vi "BM0211 Image property read write.vi"(9 "Read write":enum16{"write", "Read"}(ring)=enum."Read", 11 "IN":T1(array[cluster])) -> (0 "error out":errorcluster, 3 "Out":T1(array[cluster]))   [LabVIEW 2015]
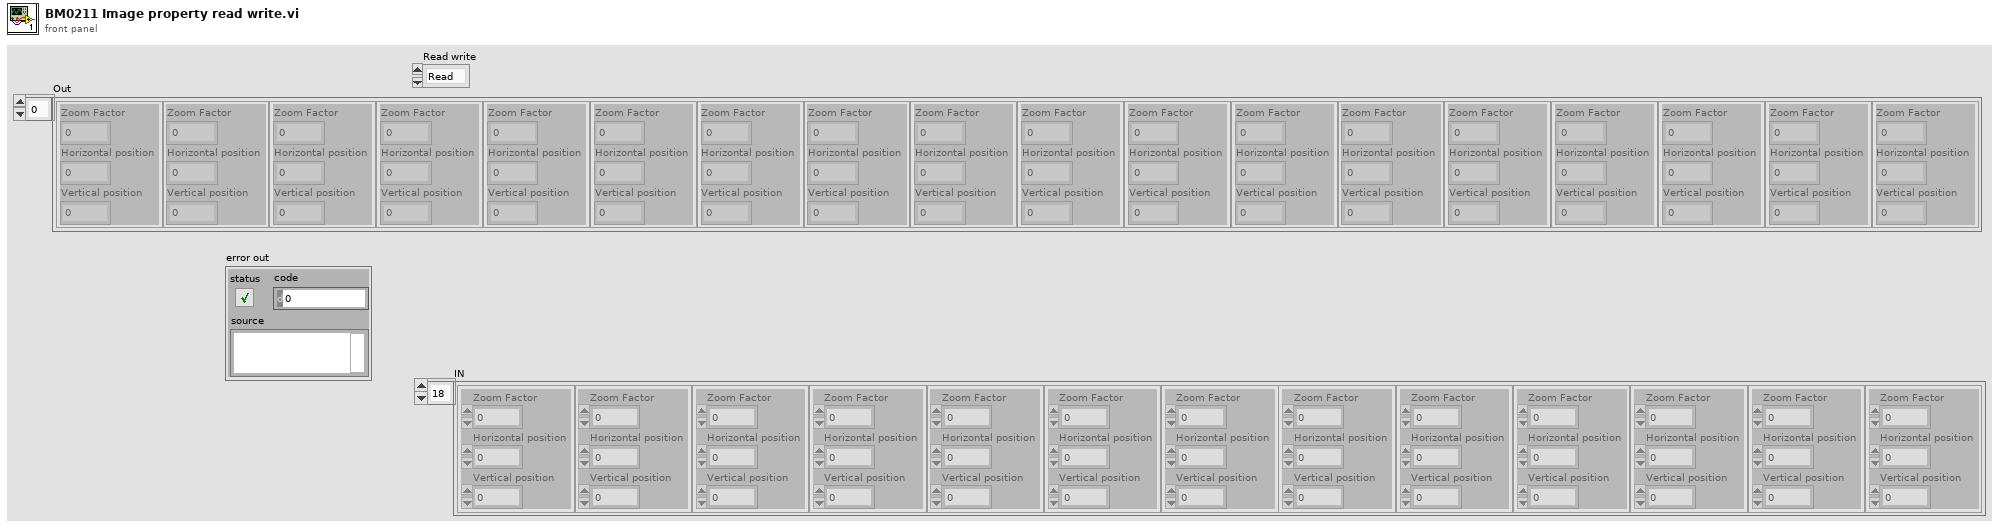
[diagram p1: front panel]
types:
  T1 = cluster{"Zoom Factor":sgl, "Horizontal position":sgl, "Vertical position":sgl}[]
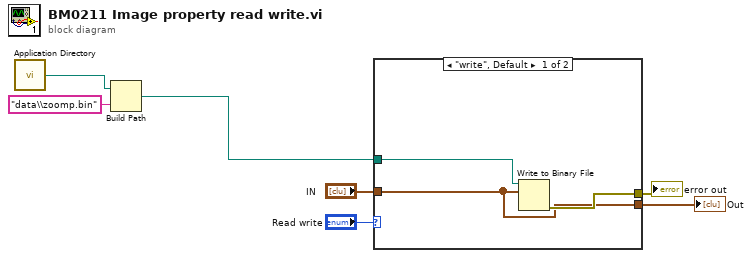
[diagram p0: block diagram]
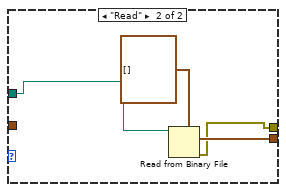
[diagram p2: hidden frame]
diagram:
  n1 = call <vilib>:"Application Directory.vi"() -> ("Application Directory"=w3:path)
  n2 = Build Path(base path=w3, name or relative path="data\\zoomp.bin") -> (appended path=w1:path)
  n3 = case shown="\"write\", Default" "Read write" {
    tunnel: "IN" -> [w8 _]
    tunnel: w1 -> [w10 w14]
    tunnel: [w8 w12] -> w5
    tunnel: [w9 w11] -> w4
    frame "write", Default {
      n4 = Write to Binary File(file (use dialog)=w10, data=w8) -> (error out=w9:errorcluster)  [unwired: 4 in, 2 out]
    }
    frame "Read" {
      n5 = Read from Binary File(5:T1 [] ("Array"), 11:w14) -> (0:w11:errorcluster, 2:w12:T1)  [unwired: 4 in, 2 out]
    }
  }
  "Out" <- w5
  "error out" <- w4
